vi "test_ConstructLabVIEWItem.vi"() -> (2 "Actuals":T1[](array[typedef]), 3 "Pass?":bool)   [LabVIEW 2020, in "Tests.LabVIEWItem.lvlib"]
uses:
  Tests.LabVIEWItem.lvlib
  Validation/Validate_BaseConstruction.ctl
  CLabVIEWItem/CLabVIEWItem.lvclass
  94520627-3d70-47dd-9449-e14d2c64ccaf.vi
  Validation/Input_BaseConstruction.ctl
  Validation/Params_ConstructLabVIEWItem.ctl
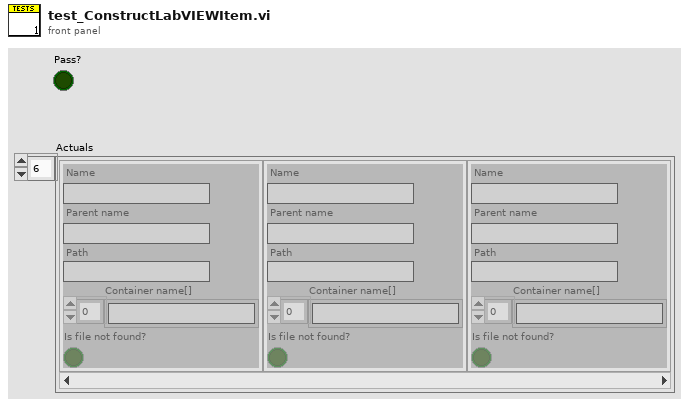
[diagram p1: front panel]
types:
  T1 = typedef "Tests.LabVIEWItem.lvlib/Validate_BaseConstruction.ctl" = cluster{"Name":string, "Parent name":string, "Path":string, "Container name[]":string[], "Is file not found?":bool}
  T2 = typedef "Tests.LabVIEWItem.lvlib/Params_ConstructLabVIEWItem.ctl" = cluster{"Input":T3, "Validation":T1}
  T3 = typedef "Tests.LabVIEWItem.lvlib/Input_BaseConstruction.ctl" = cluster{"Qualified name":string, "Path":string, "Error code":i32}
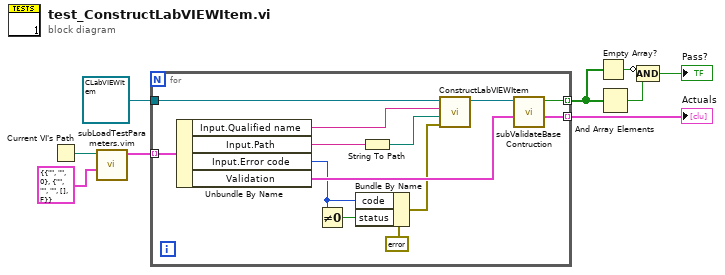
[diagram p0: block diagram]
diagram:
  n1 = Current VI's Path() -> (path=w2:path)
  n2 = call "subLoadTestParameters.vim"("Input"=T2 {"Input"={"Qualified name"="", "Path"="", "Error code"=0}, "Validation"={"Name"="", "Parent name"="", "Path"="", "Container name[]"=[], "Is file not found?"=FALSE}}, "Caller path"=w2) -> ("Params"=w1:T2[])  [unwired: 8 in, 1 out]
  n3 = for {
    tunnel: refnum<class "CLabVIEWItem.lvclass"> refnum ("CLabVIEWItem in") -> [w21]
    tunnel: [w20] -> w4 mode=indexing
    tunnel: w1 -> [w18] mode=indexing
    tunnel: [w19] -> w8 mode=indexing
    n4 = Unbundle By Name(w18) -> ("Input.Qualified name"=w16:string, "Input.Path"=w15:string, "Input.Error code"=w11:i32, "Validation"=w17:T1)
    n5 = Not Equal To 0?(x=w11) -> (x != 0?=w10:bool)
    n6 = Bundle By Name(cluster=errorcluster {"status"=FALSE, "code"=0, "source"=""} ("error in (no error)"), "code"=w11, "status"=w10) -> (w12:errorcluster)
    n7 = String To Path(string=w15) -> (path=w14:path)
    n8 = call-dynamic "ConstructLabVIEWItem.vi"("error in (no error)"=w12, "Path"=w14, "Qualified name"=w16, "CLabVIEWItem in"=w21) -> ("CLabVIEWItem out"=w22:refnum<class "CLabVIEWItem.lvclass">)  [unwired: 6 in, 1 out]
    n9 = call "subValidateBaseContruction.vi"("Parameters"=w17, "CLabVIEWItem in"=w22) -> ("Actual"=w20:T1, "Pass?"=w19:bool)  [unwired: 8 in]
  }
  "Actuals" <- w4
  n10 = Empty Array?(array=w8) -> (empty?=w7:bool)
  n11 = And Array Elements(Boolean array=w8) -> (logical AND=w6:bool)
  n12 = Compound Arithmetic op=AND(invert w7, w6) -> (→"Pass?":bool)
